vi "RT Driver VI.vi"(7 "Operation":T1, 11 "Device Reference in":T2 format="%.0x") -> (0 "Error Code":i32)   [LabVIEW 2018, in "FPGA Addon Engine.lvlib"]
uses:
  FPGA Addon Engine.lvlib
  <vilib>/NI Veristand/Custom Device API/Custom Device Item Ref.ctl
  <vilib>/NI Veristand/Custom Device API/Hardware Interface Driver VI Operation.ctl
  <vilib>/NI/NIVS Inline Async API/_VS Inline Async API/VS Inline Async API/Types/Error Handling Settings.ctl
  <vilib>/NI/NIVS Inline Async API/_VS Inline Async API/VS Inline Async API/VS Inline Async API.lvclass/VS Inline Async API.ctl
  <vilib>/NI/NIVS Inline Async API/_Data Access Engine/Data Access Engine/Data Access Engine.lvclass/Data Access Engine.ctl
  <vilib>/NI/NIVS Inline Async API/_Data Access Engine/Access Type Classes/Write/Write.lvclass/Write.ctl
  <vilib>/NI/NIVS Inline Async API/_Data Access Engine/Access Type Classes/ReadWrite/ReadWrite.lvclass/ReadWrite.ctl
  Addon Shared/SubVIs/FPGA Settings.vi
  SubVIs/Initialize Scalar Datatypes and Refs.vi
  <vilib>/NI/NIVS Inline Async API/_Data Access Engine/Data Access Engine/Methods/Data.Engine.Read Data from HW.vi
  <vilib>/NI/NIVS Inline Async API/_VS Inline Async API/Error Handling Process/SubVIs/Error.GetError.vi
  <vilib>/NI/NIVS Inline Async API/_Data Access Engine/Access Type Classes/ReadWrite/ReadWrite.EngineData.vi
  <vilib>/NI/NIVS Inline Async API/_Data Access Engine/Access Type Classes/Write/Write.EngineData.vi
  <vilib>/NI Veristand/Custom Device API/NI VeriStand - Get Channel Value by Data Reference.vi
  <vilib>/NI Veristand/Custom Device API/NI VeriStand - Set Channel Value by Data Reference.vi
  <vilib>/Utility/config.llb/Open Config Data.vi
  <vilib>/Utility/config.llb/Get Key Names.vi
  <vilib>/Utility/config.llb/Write Key.vi
  <vilib>/Utility/config.llb/Write Key (I32).vi
  <vilib>/Utility/config.llb/Close Config Data.vi
  Addon Shared/SubVIs/Constants.vi
  <vilib>/NI Veristand/Custom Device API/NI VeriStand - Get Item Property.vi
  <vilib>/NI Veristand/Custom Device API/Get Item Property (Variant).vi
  <vilib>/NI Veristand/Custom Device API/Get Item Property (Dependent File).vi
  <vilib>/NI Veristand/Custom Device API/Get Item Property (Path).vi
  <vilib>/NI Veristand/Custom Device API/Get Item Property (String).vi
  <vilib>/NI Veristand/Custom Device API/Get Item Property (Boolean).vi
  <vilib>/NI Veristand/Custom Device API/NI VeriStand - Set Item Property.vi
  <vilib>/NI Veristand/Custom Device API/Set Item Property (Path).vi
  <vilib>/NI Veristand/Custom Device API/Set Item Property (String).vi
  <vilib>/NI Veristand/Custom Device API/Set Item Property (Boolean).vi
  APIs/FPGA Register IO/Utilities/Open FPGA Session.vi
  SubVIs/Initialize Input DMA Refs.vi
  SubVIs/Initialize Output DMA Refs.vi
  SubVIs/Initialize Scalar Datatype Classes.vi
  <vilib>/Utility/SystemLogging/Write to System Log.vi
  <vilib>/Utility/error.llb/Error Cluster From Error Code.vi
  <vilib>/RVI Host/nirviSupport.llb/nirviErrorClusterFromErrorCode.vi
  <vilib>/rvi/errors/niLvFpgaAdjustHostInterfaceError.vi
  <vilib>/NI Veristand/Custom Device API/Global Data Refs.vi
  <vilib>/FPGAPlugInAG/Dynamic/niLvFpga_Close_Dynamic.vi
  <vilib>/NI Veristand/Custom Device Waveform API/Multiple Waveforms Write (DBL)/Multiple Waveforms Write (DBL).lvclass
  <vilib>/NI Veristand/Custom Device Waveform API/Single Waveform Read (DBL)/Single Waveform Read (DBL).lvclass
  <vilib>/NI/NIVS Inline Async API/_VS Inline Async API/VS Inline Async API/VS Inline Async API.lvclass
  <vilib>/rvi/interface/nirviMethod/nirviMethod.xnode
  <vilib>/rvi/interface/nirviCloseFPGA/nirviCloseFPGA.xnode
  <vilib>/NI Veristand/Custom Device API/Custom Device API.lvlib
  <vilib>/rvi/interface/nirviMethod/StockFPGA_InlinedMethodWaitForSingleIRQ.vi
  <vilib>/FPGAPlugInAG/Dynamic/niLvFpga_WaitOnIrq_Dynamic.vi
  <vilib>/FPGAPlugInAG/Dynamic/niLvFpga_AcknowledgeIrq_Dynamic.vi
  Desktop/PPL InlineTest/Source/Engine/PPL InlineTest Engine.lvlib
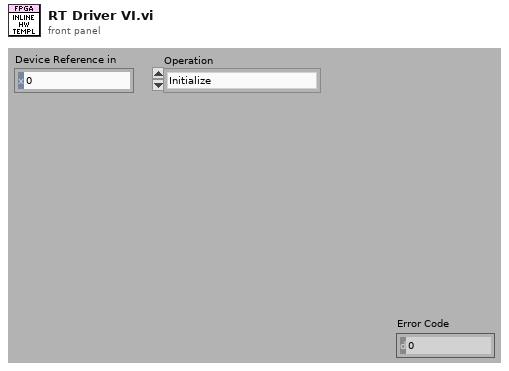
[diagram p1: front panel]
types:
  T1 = typedef "Custom Device API.lvlib/Hardware Interface Driver VI Operation.ctl" = enum16{"Initialize", "Start", "Read Data from HW", "Write Data to HW", "Close"}
  T2 = typedef "Custom Device API.lvlib/Custom Device Item Ref.ctl" = u64
  T3 = typedef "FPGA Addon Engine.lvlib/State Variables.ctl" = cluster{"FPGA Ref":refnum<k20>, "IncomingRegisters.Refs":T4[], "IncomingDMA.Refs":T7[], "OutgoingRegisters.Refs":T4[], "OutgoingDMA.Refs":T12[], "Compiled":T14}
  T4 = typedef "FPGA Addon Engine.lvlib/Register Settings.ctl" = cluster{"Name":string, "Data Type":T5, "session":u32, "Scalar Type":T6, "Index":i32, "Length":i32, "attributes":variant, "default value":variant}
  T5 = typedef "FPGA Addon Shared.lvlib/FPGA Addon Data Type.ctl" = enum8{"<Null>", "I8", "I16", "I32", "I64", "U8", "U16", "U32", "U64", "SGL", "Boolean", "Analog PWM In Settings", "Analog PWM In", "Digital PWM In Settings", "Digital PWM In", "Digital PWM Out", "Sine Out", "FXP", "FXP+/-24.5", "FXP+/-16.5", "FXP+/-32.8", "FXP+/-64.32", "FXP+/-16.7", "FXP+/-20.5", "FXP+/-27.5", "FXP+/-32.16", "FXP+16.3", "FXP+18.3", "Digital Static In", "Digital Static Out", "Digital Static In Settings", "Digital WSS Out", "Quad Encoder Settings", "Quad Encoder In", "Group"}
  T6 = typedef "FPGA Addon Shared.lvlib/Scalar Type.ctl" = enum16{"Standard", "Bitpacked"}
  T7 = typedef "FPGA Addon Engine.lvlib/DMA Input References.ctl" = cluster{"Addon Name":string, "Waveform Ref":refnum<class "Multiple Waveforms Write (DBL).lvclass">, "DMA Name":string, "DMA Settings":T8, "Refs":T11}
  T8 = typedef "FPGA Addon Shared.lvlib/DMA Settings.ctl" = cluster{"Number of Channels":u8, "Delacing Scheme":T9, "Update Rate":u32, "dt":dbl, "Mode":T10, "Number of Samples":u32, "DMA Host Buffer":u32}
  T9 = typedef "FPGA Addon Shared.lvlib/Delacing Scheme.ctl" = enum8{"Interleaved", "Bitpacked"}
  T10 = typedef "FPGA Addon Shared.lvlib/DMA Acquisition Mode.ctl" = enum8{"Continuous", "Triggered Finite"}
  T11 = typedef "FPGA Addon Engine.lvlib/DMA Input Refs.ctl" = cluster{"Data Type":T5, "DMA_SGL":refnum<k20>, "DMA_U64":refnum<k20>, "DMA_I64":refnum<k20>, "DMA_FXP+/-32.8":refnum<k20>, "DMA_FXP+/-64.32":refnum<k20>, "DMA_U32":refnum<k20>, "DMA_U16":refnum<k20>, "DMA_U8":refnum<k20>, "DMA_I32":refnum<k20>, "DMA_I16":refnum<k20>, "DMA_I8":refnum<k20>, "DMA_FXP+/-32.16":refnum<k20>}
  T12 = typedef "FPGA Addon Engine.lvlib/DMA Output References.ctl" = cluster{"Addon Name":string, "Waveforms":refnum<class "Single Waveform Read (DBL).lvclass">[], "DMA Name":string, "Refs":T13}
  T13 = typedef "FPGA Addon Engine.lvlib/DMA Output Refs.ctl" = cluster{"Data Type":T5, "DMA_SGL":refnum<k20>, "DMA_U64":refnum<k20>, "DMA_I64":refnum<k20>, "DMA_FXP+/-32.8":refnum<k20>, "DMA_FXP+/-64.32":refnum<k20>, "DMA_U32":refnum<k20>, "DMA_U16":refnum<k20>, "DMA_U8":refnum<k20>, "DMA_I32":refnum<k20>, "DMA_I16":refnum<k20>, "DMA_I8":refnum<k20>, "DMA_FXP+/-32.16":refnum<k20>}
  T14 = typedef "FPGA Addon Shared.lvlib/Compiled.Settings.ctl" = cluster{"Name":string, "IncomingRegisters.Settings":T15[], "IncomingRegisters.Refs":cluster{"Refs":T17[], "Values":dbl[]}, "OutgoingRegisters.Settings":T15[], "OutgoingRegisters.Refs":cluster{"Refs":T17[], "Values":dbl[]}, "Incoming.Size":i32, "Outgoing.Size":i32, "IncomingDMA.Settings":T19[], "OutgoingDMA.Settings":T19[], "FPGA.Settings":T21, "Target.Type":T22}
  T15 = typedef "FPGA Addon Shared.lvlib/Compiled.RegisterSettings.ctl" = cluster{"Scalar Type":T6, "Index":i32, "Length":i32, "Register":T16}
  T16 = typedef "FPGA Addon Shared.lvlib/Register Information.ctl" = cluster{"Name":string, "Data Type":T5, "Default Value":variant, "Attributes":variant}
  T17 = typedef "Custom Device API.lvlib/Block Data Reference.ctl" = cluster{"Data Reference":T18, "Offset":u64, "Length":u64}
  T18 = typedef "Custom Device API.lvlib/Data Reference.ctl" = i32
  T19 = typedef "FPGA Addon Shared.lvlib/Compiled.DMASettings.ctl" = cluster{"Name":string, "Data Type":T5, "DMA.Settings":T8, "DMA.VSRefs":T20[]}
  T20 = typedef "Custom Device API.lvlib/Waveform Data Reference.ctl" = i32
  T21 = typedef "FPGA Addon Shared.lvlib/FPGA Settings.ctl" = cluster{"Bitfile path":path, "RIO Device Address":string, "Group":bool}
  T22 = typedef "Custom Device API.lvlib/Custom Device Target Type.ctl" = enum16{"PharLap", "VxWorks", "Windows", "Linux_32_ARM", "Linux_x64"}
  T23 = cluster{"Vars":T3, "Async?":bool, "Async":refnum<class "VS Inline Async API.lvclass">}
  T24 = typedef "VS Inline Async API.lvlib/VS Inline Async API.lvclass/Error Handling Settings.ctl" = cluster{"Write to SystemLog (F)":bool}
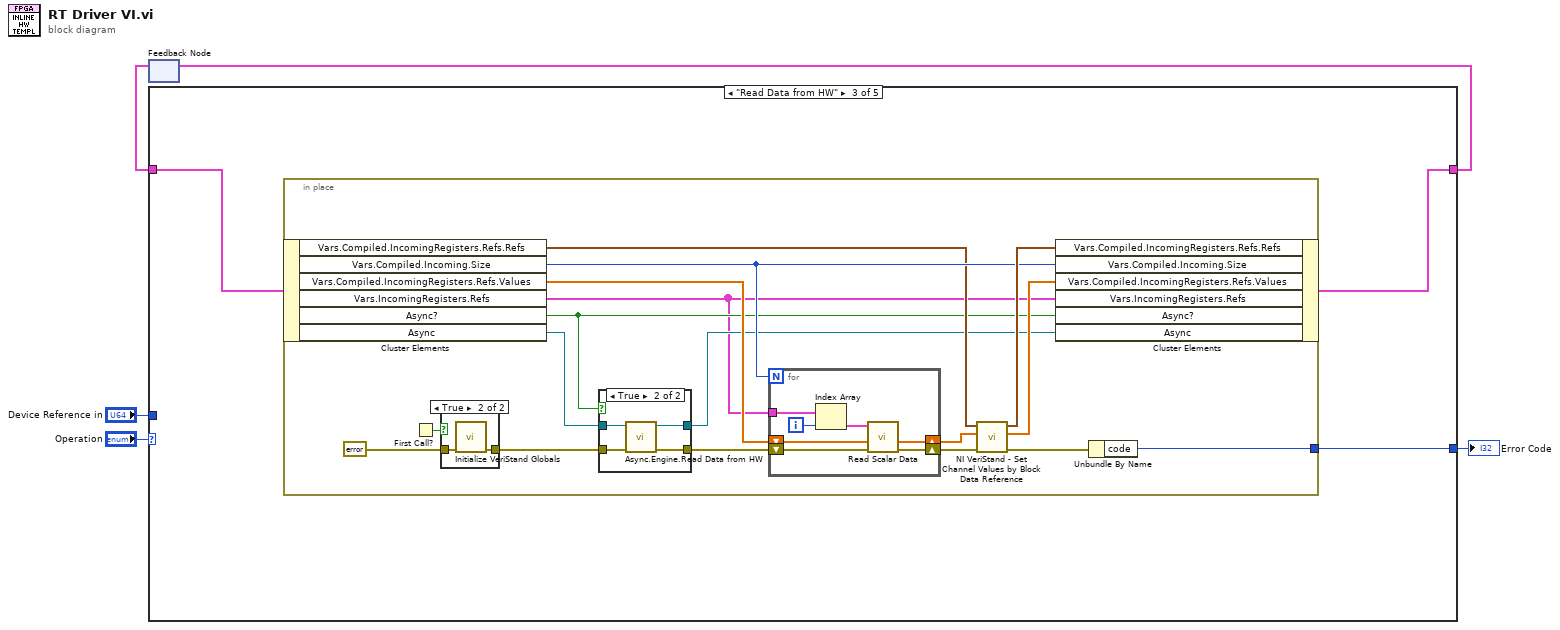
[diagram p0: block diagram]
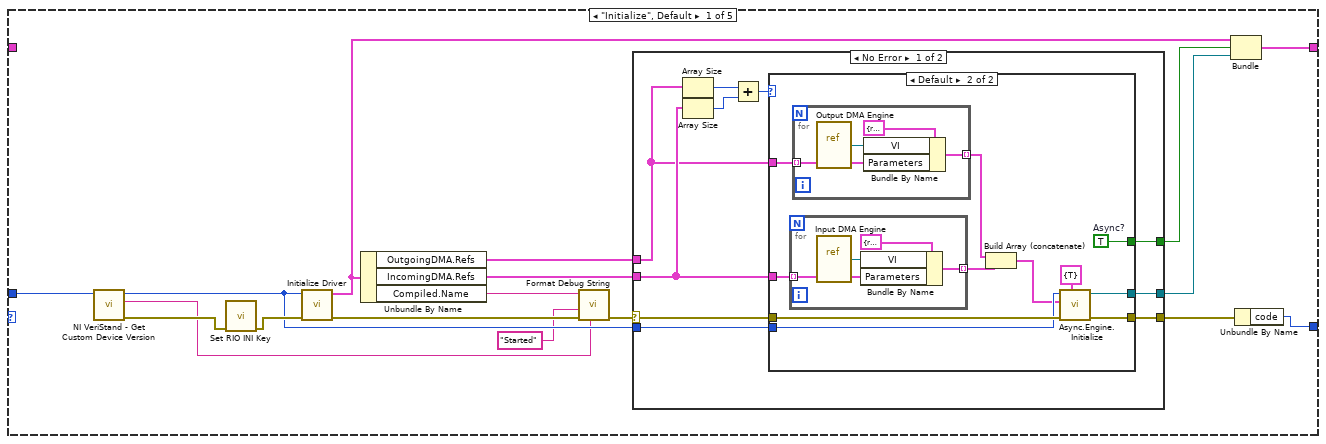
[diagram p2: hidden frame]
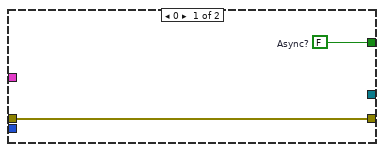
[diagram p3: hidden frame]
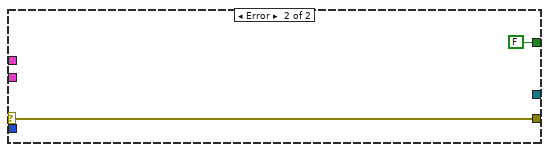
[diagram p4: hidden frame]
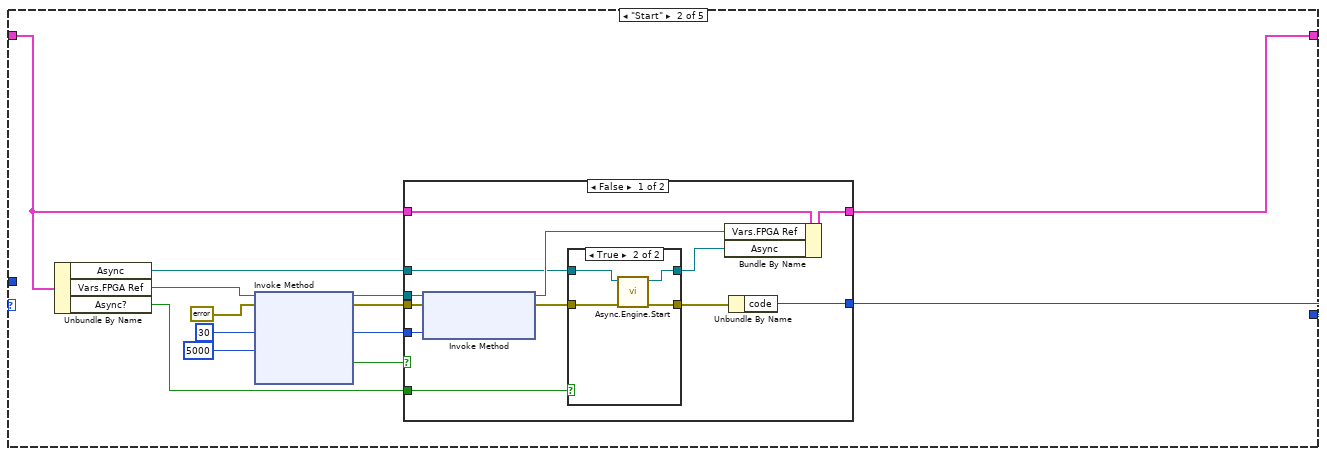
[diagram p5: hidden frame]
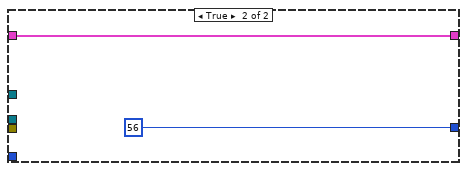
[diagram p7: hidden frame]
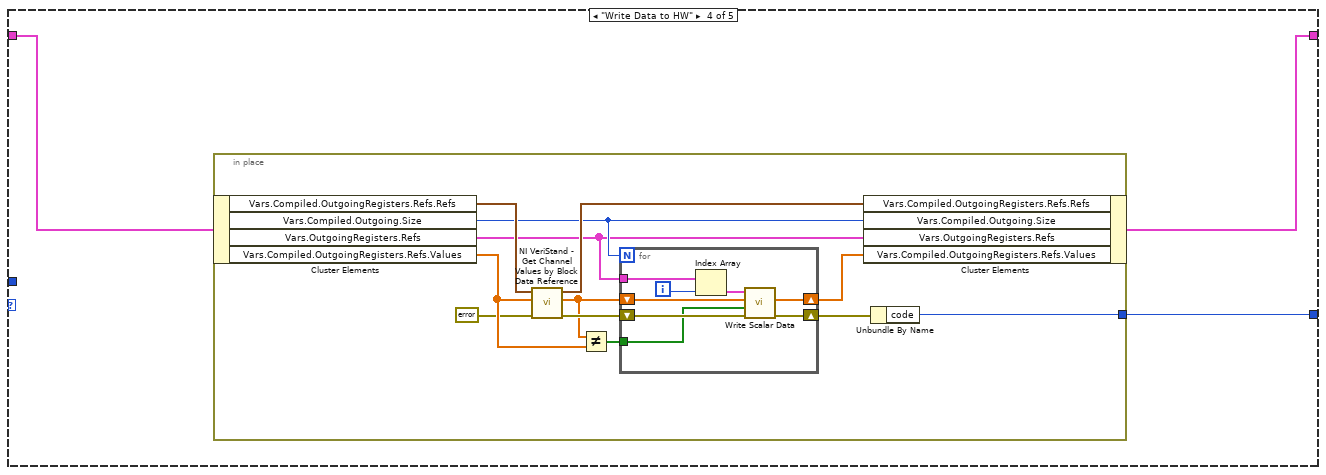
[diagram p10: hidden frame]
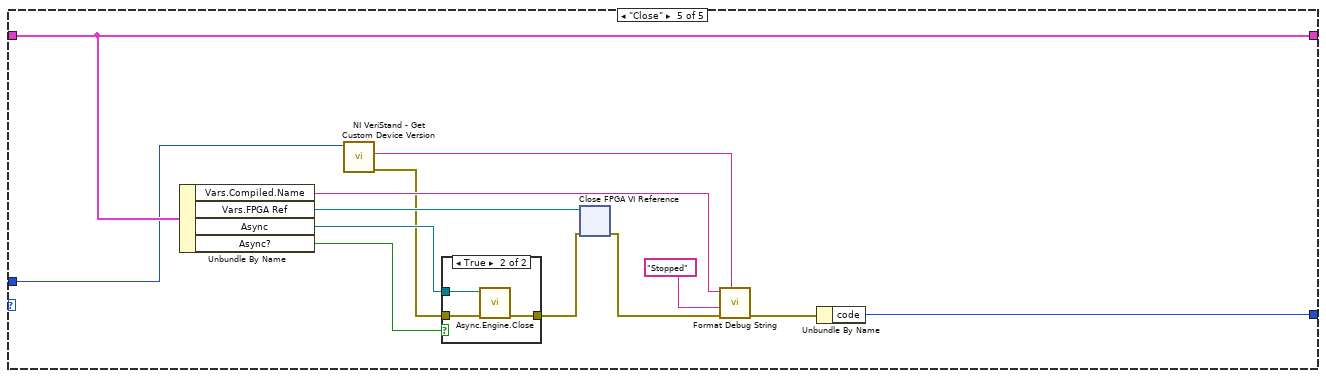
[diagram p11: hidden frame]
diagram:
  n1 = feedback #1() -> (w3:T23)  [unwired: 1 out]
  n2 = case shown="\"Read Data from HW\"" "Operation" {
    tunnel: [w22 w65 w90 w125 w158] -> w4
    tunnel: w3 -> [_ w66 w88 w126 w158]
    tunnel: "Device Reference in" -> [w12 _ _ _ w153]
    tunnel: [w21 w67 w89 w124 w159] -> w1
    frame "Initialize", Default {
      n3 = call <vilib>:"NI VeriStand - Get Custom Device Version.vi"("Device Ref in"=w12) -> ("error out"=w13:errorcluster, "Value"=w9:string, "Device Ref out"=w11:T2)  [unwired: 8 in]
      n4 = call "Set RIO INI Key.vi"("error in (no error)"=w13) -> ("error out"=w20:errorcluster)  [unwired: 10 in]
      n5 = call "Initialize Driver.vi"("error in (no error)"=w20, "Section Ref in"=w11) -> ("error out"=w10:errorcluster, "Vars"=w14:T3)  [unwired: 8 in]
      n6 = Unbundle By Name(w14) -> ("OutgoingDMA.Refs"=w16:T12[], "IncomingDMA.Refs"=w17:T7[], "Compiled.Name"=w8:string)
      n7 = call "Format Debug String.vi"("Version"=w9, "error in (no error)"=w10, "State"="Started" ("string"), "Name"=w8) -> ("error out"=w6:errorcluster)  [unwired: 7 in]
      n8 = case shown="No Error" w6 {
        selector: w6 -> [w23 w55]
        tunnel: [w32 w55] -> w19
        tunnel: [w31 _] -> w18
        tunnel: w17 -> [w30 _]
        tunnel: w16 -> [w29 _]
        tunnel: [w25 FALSE ("Async?")] -> w15
        tunnel: w11 -> [w24 _]
        frame No Error {
          n9 = Array Size(array=w29) -> (size(s)=w28:i32)
          n10 = Array Size(array=w30) -> (size(s)=w27:i32)
          n11 = Add(x=w28, y=w27) -> (x+y=w26:i32)
          n12 = case shown="Default" w26 {
            tunnel: w23 -> [w34 w42]
            tunnel: [w34 w41] -> w32
            tunnel: [_ w40] -> w31
            tunnel: w30 -> [_ w38]
            tunnel: w29 -> [_ w45]
            tunnel: [w33 w43] -> w25
            tunnel: w24 -> [_ w39]
            frame 0 {
              w33 = FALSE  # Async?
            }
            frame Default {
              w43 = TRUE  # Async?
              n13 = for {
                tunnel: w38 -> [w46] mode=indexing
                tunnel: [w48] -> w37 mode=indexing
                n14 = vi-ref "Input DMA Engine.vi"() -> (w47:refnum<vi>)
                n15 = Bundle By Name(cluster=cluster{"VI":refnum<vi>, "Parameters":variant} {"VI"=refnum, "Parameters"=variant} ("Process"), "VI"=w47, "Parameters"=w46) -> (w48:cluster{"VI":refnum<vi>, "Parameters":variant})
              }
              n16 = for {
                tunnel: w45 -> [w52] mode=indexing
                tunnel: [w51] -> w44 mode=indexing
                n17 = vi-ref "Output DMA Engine.vi"() -> (w50:refnum<vi>)
                n18 = Bundle By Name(cluster=cluster{"VI":refnum<vi>, "Parameters":variant} {"VI"=refnum, "Parameters"=variant} ("Process"), "VI"=w50, "Parameters"=w52) -> (w51:cluster{"VI":refnum<vi>, "Parameters":variant})
              }
              n19 = Build Array (concatenate)(w44, w37) -> (w36:cluster{"VI":refnum<vi>, "Parameters":variant}[])
              n20 = call <vilib>:"Async.Engine.Initialize.vi"("Error Log Settings"=T24 {"Write to SystemLog (F)"=TRUE}, "error in (no error)"=w42, "Processes"=w36, "Custom Device Ref"=w39) -> ("error out"=w41:errorcluster, "Async"=w40:refnum<class "VS Inline Async API.lvclass">)  [unwired: 6 in]
            }
          }
        }
        frame Error {
        }
      }
      n21 = Bundle("Vars"=w14, "Async?"=w15, "Async"=w18) -> (w22:T23)  [unwired: 1 out]
      n22 = Unbundle By Name(w19) -> ("code"=w21:i32)
    }
    frame "Start" {
      w61 = 30 ("IRQ Number(s)")
      n23 = Unbundle By Name(w66) -> ("Async"=w57:refnum<class "VS Inline Async API.lvclass">, "Vars.FPGA Ref"=w64:refnum<k20>, "Async?"=w59:bool)
      n24 = xnode "Invoke Method"("FPGA VI Reference In"=w64, "error in"=errorcluster {"status"=FALSE, "code"=0, "source"=""}, "IRQ Number(s)"=w61, "Timeout (ms)"=5000) -> ("FPGA VI Reference Out"=w63:refnum<k20>, "error out"=w62:errorcluster, "Timed Out"=w58:bool)  [unwired: 1 out]
      n25 = case shown="False" w58 {
        tunnel: [w79 56 ("code")] -> w67
        tunnel: w66 -> [w78 w87]
        tunnel: [w77 w87] -> w65
        tunnel: w63 -> [w76 _]
        tunnel: w62 -> [w75 _]
        tunnel: w61 -> [w74 _]
        tunnel: w59 -> [w71 _]
        tunnel: w57 -> [w70 _]
        frame False {
          n26 = xnode "Invoke Method"("FPGA VI Reference In"=w76, "error in"=w75, "IRQ Number(s)"=w74) -> ("FPGA VI Reference Out"=w73:refnum<k20>, "error out"=w68:errorcluster)
          n27 = case shown="True" w71 {
            tunnel: w68 -> [w81 w85]
            tunnel: [w81 w84] -> w72
            tunnel: w70 -> [w80 w83]
            tunnel: [w80 w82] -> w69
            frame False {
            }
            frame True {
              n28 = call <vilib>:"Async.Engine.Start.vi"("error in (no error)"=w85, "VS Inline Async API in"=w83) -> ("error out"=w84:errorcluster, "VS Inline Async API out"=w82:refnum<class "VS Inline Async API.lvclass">)  [unwired: 8 in]
            }
          }
          n29 = Bundle By Name(cluster=w78, "Vars.FPGA Ref"=w73, "Async"=w69) -> (w77:T23)
          n30 = Unbundle By Name(w72) -> ("code"=w79:i32)
        }
        frame True {
        }
      }
    }
    frame "Read Data from HW" {
      n31 = in-place {
        in-place-border: [w99] -> w89
        n32 = in-place-cluster #2(w88) -> ("Vars.Compiled.IncomingRegisters.Refs.Refs"=w101:T17[], "Vars.Compiled.Incoming.Size"=w103:i32, "Vars.Compiled.IncomingRegisters.Refs.Values"=w107:dbl[], "Vars.IncomingRegisters.Refs"=w94:T4[], "Async?"=w95:bool, "Async"=w97:refnum<class "VS Inline Async API.lvclass">)
        n33 = First Call?() -> (First Call?: T/F=w93:bool)
        n34 = case shown="True" w93 {
          tunnel: [w108 w110] -> w91
          tunnel: errorcluster {"status"=FALSE, "code"=0, "source"=""} ("error in") -> [w108 w109]
          frame False {
          }
          frame True {
            n35 = call "Initialize VeriStand Globals.vi"("error in (no error)"=w109) -> ("error out"=w110:errorcluster)  [unwired: 10 in]
          }
        }
        n36 = case shown="True" w95 {
          tunnel: w97 -> [w112 w116]
          tunnel: [w111 w115] -> w98
          tunnel: [w112 w114] -> w96
          tunnel: w91 -> [w111 w113]
          frame False {
          }
          frame True {
            n37 = call <vilib>:"Async.Engine.Read Data from HW.vi"("error in"=w113, "Async in"=w116) -> ("error out"=w115:errorcluster, "Async out"=w114:refnum<class "VS Inline Async API.lvclass">)  [unwired: 8 in]
          }
        }
        n38 = for {
          N: w103 -> [_]
          shift-right: [w117] -> w104
          shift-left: w107 -> [w118]
          shift-right: [w121] -> w102
          shift-left: w98 -> [w122]
          tunnel: w94 -> [w123]
          i -> [w119]
          n39 = Index Array(array=w123, index=w119) -> (element=w120:T4)
          n40 = call "Read Scalar Data.vi"("error in (no error)"=w122, "Values"=w118, "Cluster"=w120) -> ("error out"=w121:errorcluster, "Values"=w117:dbl[])  [unwired: 7 in]
        }
        n41 = call <vilib>:"NI VeriStand - Set Channel Values by Block Data Reference.vi"("error in (no error)"=w102, "Values Array in"=w104, "Block Data Ref"=w101) -> ("error out"=w100:errorcluster, "Values Array out"=w105:dbl[], "Block Data Ref dup"=w106:T17[])  [unwired: 6 in]
        n42 = in-place-cluster #2("Vars.Compiled.IncomingRegisters.Refs.Refs"=w106, "Vars.Compiled.Incoming.Size"=w103, "Vars.Compiled.IncomingRegisters.Refs.Values"=w105, "Vars.IncomingRegisters.Refs"=w94, "Async?"=w95, "Async"=w96) -> (w90:T23)
        n43 = Unbundle By Name(w100) -> ("code"=w99:i32)
      }
    }
    frame "Write Data to HW" {
      n44 = in-place {
        in-place-border: [w132] -> w124
        n45 = in-place-cluster #3(w126) -> ("Vars.Compiled.OutgoingRegisters.Refs.Refs"=w138:T17[], "Vars.Compiled.Outgoing.Size"=w134:i32, "Vars.OutgoingRegisters.Refs"=w127:T4[], "Vars.Compiled.OutgoingRegisters.Refs.Values"=w130:dbl[])
        n46 = call <vilib>:"NI VeriStand - Get Channel Values by Block Data Reference.vi"("error in (no error)"=errorcluster {"status"=FALSE, "code"=0, "source"=""} ("error in"), "Values Array in"=w130, "Block Data Ref"=w138) -> ("error out"=w135:errorcluster, "Values Array out"=w131:dbl[], "Block Data Ref dup"=w137:T17[])  [unwired: 6 in]
        n47 = Not Equal?(x=w131, y=w130) -> (x != y?=w129:bool[])
        n48 = for {
          N: w134 -> [_]
          shift-right: [w140] -> w136
          shift-left: w131 -> [w145]
          shift-right: [w141] -> w133
          shift-left: w135 -> [w146]
          tunnel: w129 -> [w139]
          tunnel: w127 -> [w144]
          i -> [w142]
          n49 = Index Array(array=w144, index=w142) -> (element=w143:T4)
          n50 = call "Write Scalar Data.vi"("error in (no error)"=w146, "Changed?"=w139, "Values"=w145, "Cluster"=w143) -> ("error out"=w141:errorcluster, "Values"=w140:dbl[])  [unwired: 6 in]
        }
        n51 = in-place-cluster #3("Vars.Compiled.OutgoingRegisters.Refs.Refs"=w137, "Vars.Compiled.Outgoing.Size"=w134, "Vars.OutgoingRegisters.Refs"=w127, "Vars.Compiled.OutgoingRegisters.Refs.Values"=w136) -> (w125:T23)
        n52 = Unbundle By Name(w133) -> ("code"=w132:i32)
      }
    }
    frame "Close" {
      n53 = Unbundle By Name(w158) -> ("Vars.Compiled.Name"=w148:string, "Vars.FPGA Ref"=w156:refnum<k20>, "Async"=w154:refnum<class "VS Inline Async API.lvclass">, "Async?"=w155:bool)
      n54 = call <vilib>:"NI VeriStand - Get Custom Device Version.vi"("Device Ref in"=w153) -> ("error out"=w147:errorcluster, "Value"=w149:string)  [unwired: 8 in, 1 out]
      n55 = case shown="True" w155 {
        tunnel: [w160 w163] -> w157
        tunnel: w154 -> [_ w162]
        tunnel: w147 -> [w160 w161]
        frame False {
        }
        frame True {
          n56 = call <vilib>:"Async.Engine.Close.vi"("error in (no error)"=w161, "Async in"=w162) -> ("error out"=w163:errorcluster)  [unwired: 8 in, 1 out]
        }
      }
      n57 = xnode "Close FPGA VI Reference"("FPGA VI Reference In"=w156, "error in"=w157) -> ("error out"=w150:errorcluster)
      n58 = call "Format Debug String.vi"("Version"=w149, "error in (no error)"=w150, "State"="Stopped" ("string"), "Name"=w148) -> ("error out"=w151:errorcluster)  [unwired: 7 in]
      n59 = Unbundle By Name(w151) -> ("code"=w159:i32)
    }
  }
  "Error Code" <- w1
  n60 = feedback-in #1(w4) -> ()
